vi "Remove.vi"(8 "error in (no error)":errorcluster, 10 "Index":i32, 11 "ListImp in":refnum<class "ListImp.lvclass">) -> (0 "error out":errorcluster, 1 "Item":refnum<class>, 3 "ListImp out":refnum<class "ListImp.lvclass">)   [LabVIEW 2017, in "LapDog.Collections.v0.Lists.lvlib" / "ListImp.lvclass"]
uses:
  ListImp.lvclass
  ListImp.lvclass/ListImp.ctl
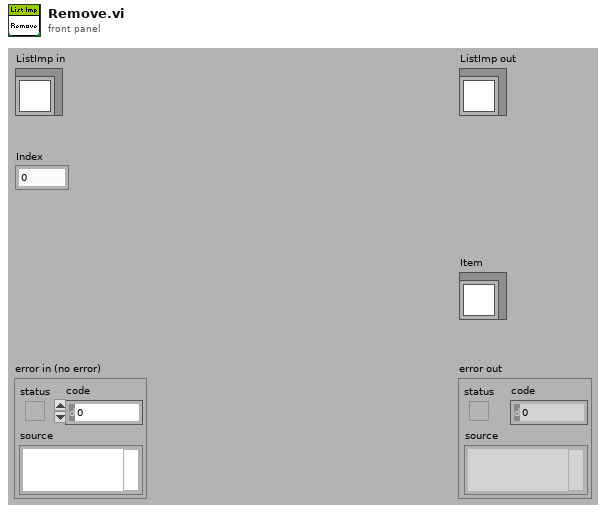
[diagram p1: front panel]
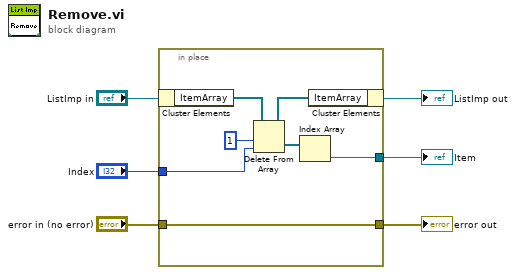
[diagram p0: block diagram]
diagram:
  n1 = in-place {
    in-place-border: "error in (no error)" -> [w13]
    in-place-border: [w13] -> w5
    in-place-border: [w12] -> w2
    in-place-border: "Index" -> [w11]
    n2 = in-place-cluster #1("ListImp in") -> ("ItemArray"=w10:refnum<class>[])
    n3 = Delete From Array(array=w10, length=1, index=w11) -> (deleted portion=w7:refnum<class>[], array with subset deleted=w9:refnum<class>[])
    n4 = Index Array(array=w7) -> (element=w12:refnum<class>)  [unwired: 1 in]
    n5 = in-place-cluster #1("ItemArray"=w9) -> (→"ListImp out":refnum<class "ListImp.lvclass">)
  }
  "error out" <- w5
  "Item" <- w2
